vi "01_splitter.vi"(11 "String":string) -> (3 "Array":string[](array[string]))   [LabVIEW 2019]
panel:
  out "offset past token":i32
  out "remaining string":string
  out "output 1":string
  out "Numeric":i32
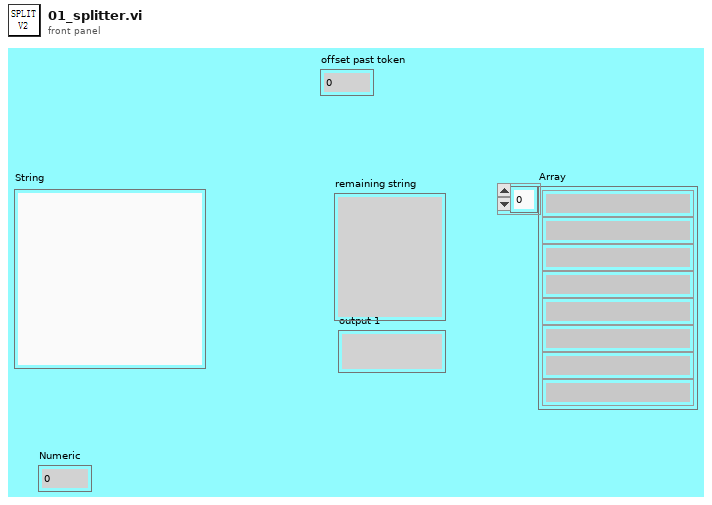
[diagram p1: front panel]
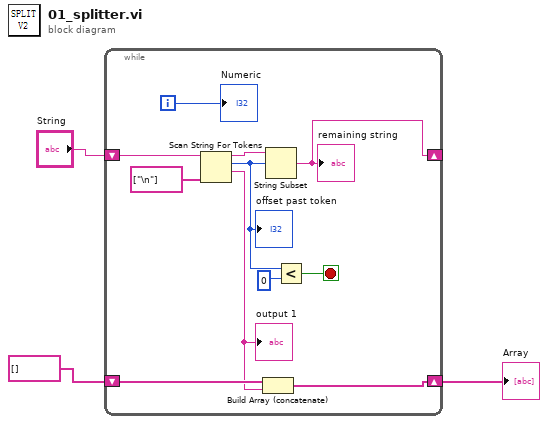
[diagram p0: block diagram]
diagram:
  n1 = while {
    shift-right: [w8] -> _
    shift-left: "String" -> [w11]
    shift-right: [w12] -> w1
    shift-left: string[] [] -> [w13]
    i -> [w14]
    stop <- w5 stop-if-true
    n2 = Scan String For Tokens(6:string[] ["\n"] ("delimiters (\\s,\\t,\\r,\\n)"), 9:w11) -> (1:w4:string, 2:w7:i32, 3:w9:string)  [unwired: 4 in, 1 out]
    "output 1" <- w4
    "offset past token" <- w7
    n3 = Build Array (concatenate)(w13, w4) -> (w12:string[])
    n4 = String Subset(string=w9, offset (0)=w7) -> (substring=w8:string)  [unwired: 1 in]
    "remaining string" <- w8
    n5 = Less?(x=w7, y=0) -> (x < y?=w5:bool)
    "Numeric" <- w14
  }
  "Array" <- w1
